vi "GetLimsTestsForBench.vi"(8 "error in (no error)":errorcluster, 10 "Data in":T1, 11 "ByteGSAPIBase in":refnum<class "ByteGSAPIBase.lvclass">) -> (0 "error out":errorcluster, 2 "Tests for bench":T2[](array[typedef]), 3 "ByteGSAPIBase out":refnum<class "ByteGSAPIBase.lvclass">)   [LabVIEW 2019, in "ByteGSWebAPI.lvlib" / "ByteGSAPIBase.lvclass"]
doc: "Richiesta lista dei Test in base alla Postazione e la Data (opzionale)"
uses:
  ByteGSAPIBase.lvclass
  TypeDef/Test.ctl
  TypeDef/Asset.ctl
  ByteGSAPIBase.lvclass/ByteGSAPIBase.ctl
  <vilib>/Bytelabs/ByteREST/ByteRESTClass/ByteRESTBase/RESTBase.lvclass
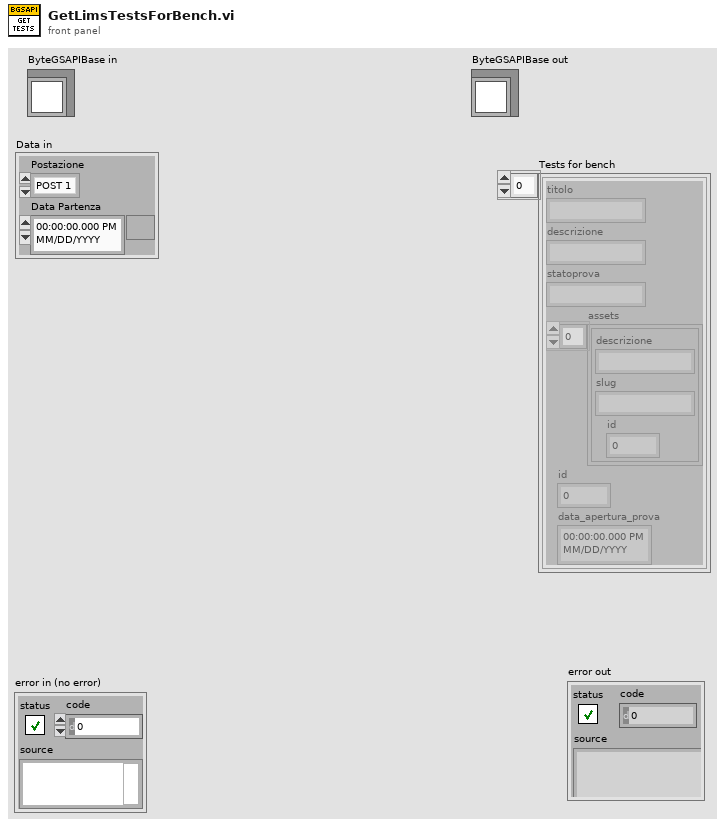
[diagram p1: front panel]
types:
  T1 = cluster{"Postazione":enum16{"POST 1", "POST 2"}, "Data Partenza":timestamp}
  T2 = typedef "ByteGSWebAPI.lvlib/ByteGSAPIBase.lvclass/Test.ctl" = cluster{"titolo":string, "descrizione":string, "statoprova":string, "assets":T3[], "id":i32, "data_apertura_prova":timestamp}
  T3 = typedef "ByteGSWebAPI.lvlib/ByteGSAPIBase.lvclass/Asset.ctl" = cluster{"descrizione":string, "slug":string, "id":i32}
  T4 = cluster{"titolo":string, "descrizione":string, "statoprova":string, "assets":cluster{"descrizione":string, "slug":string, "id":i32}[], "data_apertura_prova":string, "id":i32}[]
  T5 = cluster{"descrizione":string, "slug":string, "id":i32}[]
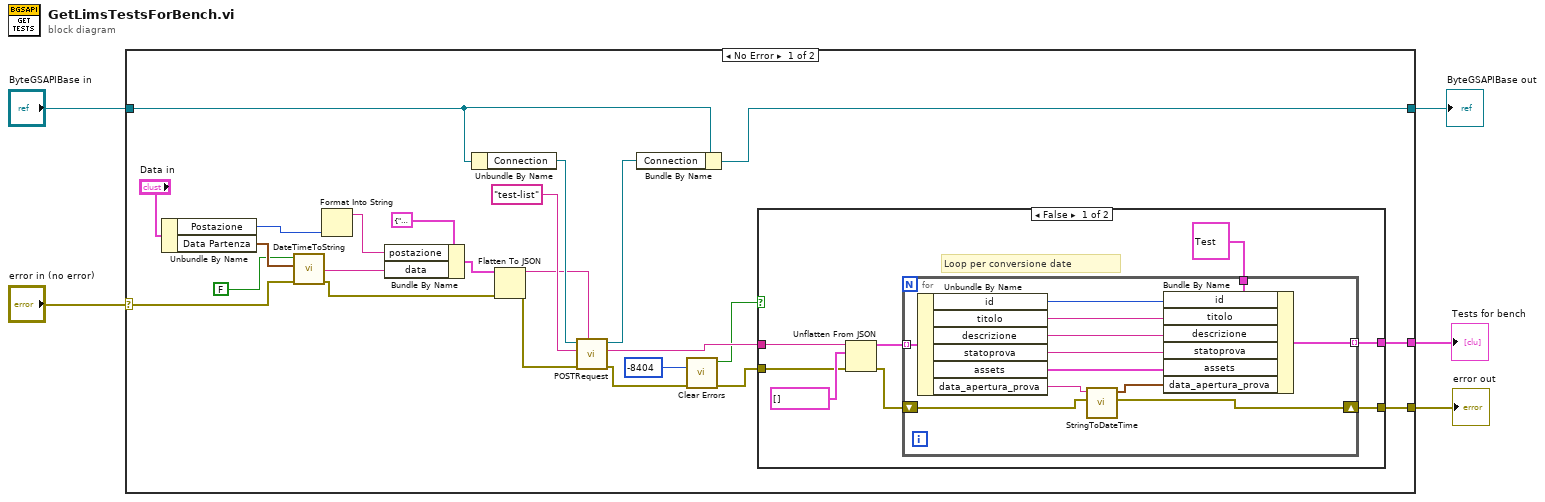
[diagram p0: block diagram]
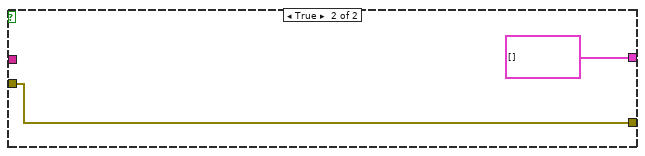
[diagram p2: hidden frame]
diagram:
  n1 = case shown="No Error" "error in (no error)" {
    selector: "error in (no error)" -> [w12 w53]
    tunnel: [w22 w53] -> w4
    tunnel: [w27 w52] -> w2
    tunnel: "ByteGSAPIBase in" -> [w20 w52]
    tunnel: [w21 _] -> w1
    frame No Error {
      n2 = Unbundle By Name("Data in") -> ("Postazione"=w14:enum16{"POST 1", "POST 2"}, "Data Partenza"=w18:timestamp)
      n3 = call "DateTimeToString.vi"("error in"=w12, "current time"=w18, "Time"=FALSE) -> ("error out"=w13:errorcluster, "Date string"=w11:string)  [unwired: 7 in]
      n4 = Format Into String(w14) -> (resulting string=w15:string)  [unwired: 3 in, 1 out]
      n5 = Bundle By Name(cluster=cluster{"postazione":string, "data":string} {"postazione"="", "data"=""} ("Request"), "postazione"=w15, "data"=w11) -> (w16:cluster{"postazione":string, "data":string})
      n6 = Unbundle By Name(w20) -> ("Connection"=w29:refnum<class "RESTBase.lvclass">)
      n7 = Flatten To JSON(anything=w16, error in (no error)=w13) -> (JSON string=w25:string, 11:w24:errorcluster)  [unwired: 1 in]
      n8 = call-dynamic "POSTRequest.vi"("Body in"=w25, "error in (no error)"=w24, "Request"="test-list", "ByteRESTBase in"=w29) -> ("error out"=w8:errorcluster, "Body"=w23:string, "ByteRESTBase out"=w28:refnum<class "RESTBase.lvclass">)  [unwired: 4 in, 1 out]
      n9 = Bundle By Name(cluster=w20, "Connection"=w28) -> (w27:refnum<class "ByteGSAPIBase.lvclass">)
      n10 = call <vilib>:"Clear Errors.vi"("error in (no error)"=w8, "specific error code to clear (0: all)"=-8404) -> ("error out"=w7:errorcluster, "specific error cleared?"=w6:bool)  [unwired: 4 in]
      n11 = case shown="False" w6 {
        tunnel: w23 -> [w37 _]
        tunnel: [w33 w51] -> w22
        tunnel: [w32 T2[] []] -> w21
        tunnel: w7 -> [w30 w51]
        frame False {
          # "Loop per conversione date"
          n12 = Unflatten From JSON(JSON string=w37, type and defaults=T4 [], error in (no error)=w30) -> (value=w35:T4, error out=w34:errorcluster)  [unwired: 4 in]
          n13 = for {
            tunnel: w35 -> [w49] mode=indexing
            tunnel: T2 {"titolo"="", "descrizione"="", "statoprova"="", "assets"=[], "id"=0, "data_apertura_prova"=timestamp(0 s since 1904-01-01)} ("ByteGSWebAPI.lvlib:ByteGSAPIBase.lvclass:Test") -> [w48]
            shift-right: [w38] -> w33
            shift-left: w34 -> [w39]
            tunnel: [w42] -> w32 mode=indexing
            n14 = Unbundle By Name(w49) -> ("id"=w47:i32, "titolo"=w46:string, "descrizione"=w45:string, "statoprova"=w44:string, "assets"=w43:T5, "data_apertura_prova"=w41:string)
            n15 = call "StringToDateTime.vi"("error in (no error)"=w39, "datetime string"=w41) -> ("error out"=w38:errorcluster, "timestamp"=w40:timestamp)  [unwired: 8 in]
            n16 = Bundle By Name(cluster=w48, "id"=w47, "titolo"=w46, "descrizione"=w45, "statoprova"=w44, "assets"=w43, "data_apertura_prova"=w40) -> (w42:T2)
          }
        }
        frame True {
        }
      }
    }
    frame Error {
    }
  }
  "error out" <- w4
  "ByteGSAPIBase out" <- w2
  "Tests for bench" <- w1
